vi "Get Services JSON Path.vi"(8 "error in (no error)":errorcluster) -> (0 "error out":errorcluster, 1 "path exists":bool, 2 "services root directory":path, 3 "services JSON path":path)   [LabVIEW 2021, in "NI Discovery V1 Client.lvlib"]
uses:
  NI Discovery V1 Client.lvlib
  <vilib>/Utility/sysdir.llb/System Directory Type.ctl
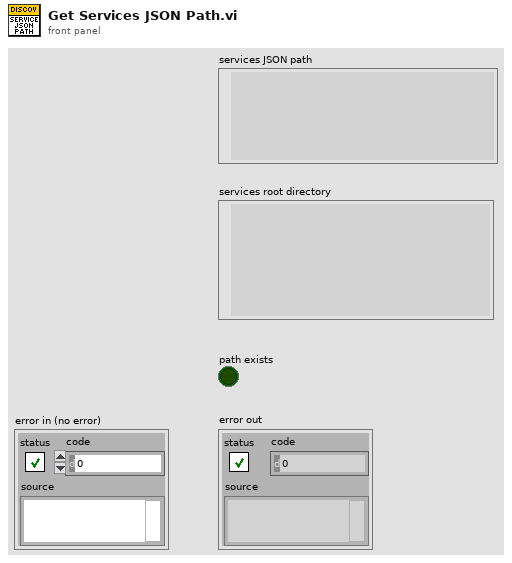
[diagram p1: front panel]
types:
  T1 = typedef "System Directory Type.ctl" = i32
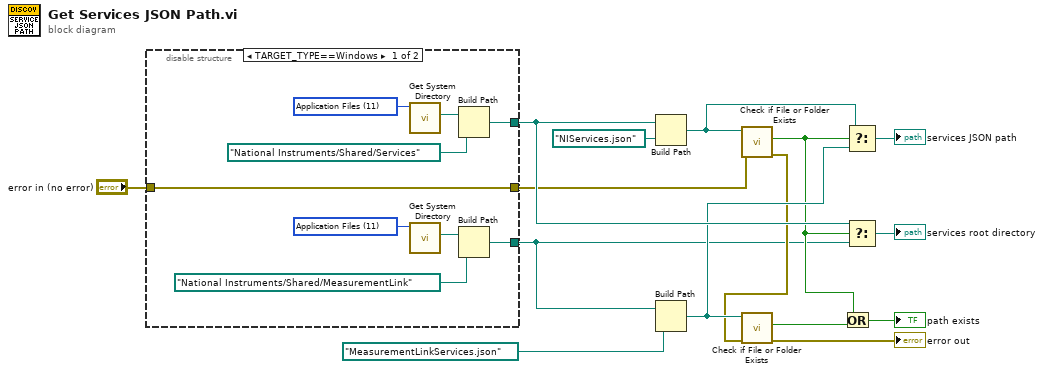
[diagram p0: block diagram]
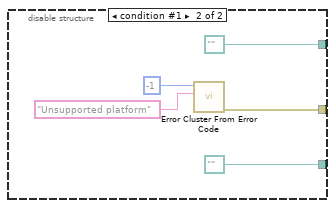
[diagram p2: hidden frame]
diagram:
  n1 = disable-structure shown="TARGET_TYPE==Windows" {
    disable-tunnel: [w21 path "" ("appended path")] -> w12
    disable-tunnel: "error in (no error)" -> [w20 _]
    disable-tunnel: [w20 w27] -> w2
    disable-tunnel: [w16 path "" ("appended path")] -> w1
    frame condition #0 (active) {
      w19 = T1 11 items=["User Home"=0, "User Desktop"=1, "User Documents"=2, "User Application Data"=3, "User Preferences"=4, "User Temporary"=5, "Public Documents"=6, "Public Application Data"=7, "Public Preferences"=8, "Public Cache"=13, "System Core Libraries"=9, "System Installed Libraries"=10, "Application Files"=11, "Boot Volume Root"=12] ("system directory type")
      w24 = T1 11 items=["User Home"=0, "User Desktop"=1, "User Documents"=2, "User Application Data"=3, "User Preferences"=4, "User Temporary"=5, "Public Documents"=6, "Public Application Data"=7, "Public Preferences"=8, "Public Cache"=13, "System Core Libraries"=9, "System Installed Libraries"=10, "Application Files"=11, "Boot Volume Root"=12] ("system directory type")
      n2 = call <vilib>:"Get System Directory.vi"("system directory type"=w24) -> ("system directory"=w23:path)  [unwired: 10 in]
      n3 = call <vilib>:"Get System Directory.vi"("system directory type"=w19) -> ("system directory"=w18:path)  [unwired: 10 in]
      n4 = Build Path(base path=w23, name or relative path=path "National Instruments/Shared/Services") -> (appended path=w21:path)
      n5 = Build Path(base path=w18, name or relative path=path "National Instruments/Shared/MeasurementLink") -> (appended path=w16:path)
    }
    frame condition #1 {
      n6 = call <vilib>:"Error Cluster From Error Code.vi"("error message (\"\")"="Unsupported platform" ("error message (\"\")"), "error code (0)"=-1) -> ("error out"=w27:errorcluster)  [unwired: 7 in]
    }
  }
  n7 = Build Path(base path=w12, name or relative path=path "NIServices.json") -> (appended path=w13:path)
  n8 = Build Path(base path=w1, name or relative path=path "MeasurementLinkServices.json") -> (appended path=w9:path)
  n9 = call <vilib>:"Check if File or Folder Exists.vi"("error in (no error)"=w2, "path"=w13) -> ("error out"=w8:errorcluster, "file or folder exists?"=w6:bool)  [unwired: 7 in, 1 out]
  n10 = call <vilib>:"Check if File or Folder Exists.vi"("error in (no error)"=w8, "path"=w9) -> ("error out"=→"error out":errorcluster, "file or folder exists?"=w5:bool)  [unwired: 7 in, 1 out]
  n11 = Or(x=w6, y=w5) -> (x .or. y?=→"path exists":bool)
  n12 = Select(t=w13, s=w6, f=w9) -> (s? t:f=→"services JSON path":path)
  n13 = Select(t=w12, s=w6, f=w1) -> (s? t:f=→"services root directory":path)
